vi "RTHeader.vi"(0 "Comment":string, 1 "Digitizer Settings":T10={"Digitizer delay (us) "=0.0, "rf points per line"=2048, "lines per plane"=128, "Samp Rate (Hz)"=100000000.0, "Additional dig delay (us)"=0.0, "Voltage Scale"=0.4, "Pre-Looks"=0, "Offset delay (us)"=0.0, "bits A/D"=8, "Avg Num"=1, "DigTimeOut"=5.0, "Rel Dig Delay"=0.0, "Dig Ch"=0, "LeCroyCluster"={"LeCroy Channels"=[TRUE, FALSE, FALSE, FALSE], "LC read pt offset"=0.0, "Sweep Avg"=FALSE}, "Main Digitizer"=enum."NI Digitizer", "Dig Config"=enum."Single channel", "Digitizer ID Cluster"={"Acqiris/Alazar/SP ID"=[], "NI Instr Handles"=[], "LeCroy VISA"="", "GaGe Handle"={"Handle"=0, "Sample size"=0, "Resolution"=0, "Offset"=0, "Channels"=0, "Boards"=0}, "ATS Ref"="ATS9350", "Acqiris Address"=["PCI::INSTR0"], "ADQRef"=refnum, "adq_cu_ptr"=refnum}, "Trigger Settings"={"Trig Source"=1, "Trig Coupling"=0, "Trig Slope"=0, "Level (mV)"=1500.0}, "Bulk Acq"=FALSE, "Bulk Start Indexes"=[], "Data Ref RF"=refnum, "NI ID/Channel"=[], "Total Dig CH"=1, "Xtra Ann Trig delay (us)"=10.0, "Fix Z Delay?"=FALSE, "One Way Transmission?"=FALSE, "Data Ref Log"=refnum} {"Trigger Settings"."Trig Slope" items=["Positive", "Negative"]; "Trigger Settings"."Level (mV)" format="%.2f"; "Trigger Settings"."Trig Coupling" items=["DC 1 MOhm", "AC 1 MOhm", "DC 50 Ohm", "AC 50 Ohm"]; "Trigger Settings"."Trig Source" items=["Chan 1", "External"]; "Rel Dig Delay" format="%.2f"; "DigTimeOut" format="%.2f"; "Avg Num" min=1; "Offset delay (us)" format="%.2f"; "Additional dig delay (us)" format="%.2f"; "Digitizer delay (us)" format="%.2f"}, 3 "Dig Word Size":u16=8, 5 "File Name In":string, 7 "Patient Info":T1={"Eye Selector"=enum."Right", "Plane"=1, "First Name"="", "Last Name"="", "Notes"="", "Patient ID"="", "Scan Location"=enum."Radio Selection 1"} {"Plane" min=1 max=12 step=1 scale=0.0..12.0}, 9 "Ann Array Params":T2={"Synth Foc?"=FALSE, "Focal Zones"=41, "Switch T/R"=0, "Trans Geometry (mm)"={"Transducer"=0, "Geo Focus"=12.0, "a (radius)"=3.0, "# of rings"=5, "kerf space "=0.1, "Center Freq"=12.0}, "Sub Ap Excite?"=FALSE, "Full Array Scan?"=FALSE, "Xmt/Rcv"={"XMIT"=[TRUE, TRUE, TRUE, TRUE, TRUE], "RCV"=[TRUE, TRUE, TRUE, TRUE, TRUE]}, "PulseSpacing (us)"=0.0, "Xmit Ring"=0, "XMIT CHS"=0, "RCV CHS"=0, "GPU?"=FALSE, "Save TIFF?"=FALSE, "downfactor"=1, "RCV 1CH"=0} {"RCV 1CH" items=["All", "1", "2", "3", "4", "5"]; "Trans Geometry (mm)"."Transducer" items=["6D 12R 40 MHz"=0, "10D 31R 20 MHz"=1, "10D 23R 20 MHz"=2, "6D 23R 40 MHz"=3, "4.5D 10.7R 40 MHz"=4, "9D 23.5R 20 MHz"=5, "9D 25.8R 20MHz"=6, "Enter"=99]; "Switch T/R" min=1 max=5 step=1}, 11 "Votage scaling":T15, 12 "Pulser Channel":i32, 14 "Scan Info":T5, 15 "Motion Settings":T6={"No Motion?"=FALSE, "Motion System"=enum."NI 735x", "Motion Bd ID"=1, "Motion Profile"="SMAC1", "# Axis"=1, "Reverse Z axis?"=TRUE, "SMAC Axis"=0, "scan pair"=enum."y-(x) scan", "RT fps"=6.0, "Steps per mm"=[1000, 1000, 1000, 1000], "Motor Parameters"={"velocity ct/s"=[10000.0, 10000.0, 10000.0, 50000.0], "accel ct/s^2"=[50000.0, 50000.0, 50000.0, 200000.0]}, "One Way Scan"=FALSE, "Reverse One Way Scan"=FALSE, "Global Position (mm)"=[], "Plane"=0, "Distance between\nscan lines (um)"=0.0, "Distance between\nscan planes (um)"=0.0, "number of scan planes"=1, "Total steps in line"=0, "Xtra plane\ndistance  (um)"=100, "Xtra planes "=1, "Add Axis"=FALSE, "overshoot cts"=200, "BKPT Shift"=0, "Scan Start Time (ms)"=0, "ESP VISA"="GPIB::1::INSTR", "3rd Axis"=1, "GL Ref Out"=refnum, "Galil Address"=""} {"3rd Axis" items=["x", "y", "z", "w"]; "Xtra planes" min=1; "Xtra plane\ndistance  (um)" min=0; "Distance between\nscan planes (um)" format="%.2f"; "Distance between\nscan lines (um)" format="%.2f"; "SMAC Axis" items=["None"=0, "Axis 1"=1, "Axis 2"=2, "Axis 3"=3, "Axis 4"=4, "Axis 5"=5, "Axis 6"=6, "Axis 7"=7, "Axis 8"=8, "Vector Space 1"=17, "Vector Space 2"=18, "Vector Space 3"=19, "Vector Space 4"=20]; "Motion Bd ID" min=1 max=32 step=1}) -> (4 "Header String Out":string, 10 "Header Out":T14={"header info"={"Header"="", "Head length"=0}, "A/D info"={"# rf points per line"=0, "# lines per scan"=0, "sample rate MHz"=0, "# A/D bits"=0, "# bytes per A/D"=0, "TGC Flag"=0, "A/D Type"=""}, "Tranducer Info"={"bandwidth"=0.0, "center freq"=0.0, "start freq"=0.0, "ID"=0}, "Scan Info"={"delay"=0.0, "pivot distance"=0.0, "sector scan angle"=0.0, "operator"="", "Scan Mode"="", "location"=""}, "Time/Date Info"={"date"="", "time"=""}, "RF Info"={"RF file name"="", "RF file att"="", "RF cal file name"="", "RF cal file att"=""}, "Patient Info"={"ID"="", "extended ID"="", "age"=0, "sex"="", "previously\nscanned"="", "PSA"=0.0, "LOS"=1, "Ethnicty 2"=3, "Race"=3}, "Tissue Type"={"organ"=0, "disease type"=0, "disease location"=0, "IQ_pts"=0, "RcvBuffer"=0, "RcvFrame"=0, "IQBuff"=0, "IQFrame"=0, "IQPage"=0}, "Votage scaling"={"Digitizer (dB)"=0.0, "Gain (dB)"=0.0, "Atten (dB)"=0.0}, "Comment"="", "Misc Info"={"avg num"=0, "c speed"=0, "Div By or SF zones"=0, "XMIT CHS"=0, "RCV CHS"=0, "Xmit angle"=0.0}, "Therapy Parameters"={"Theraputic Freq (MHz)"=0.1, "Time on (s)"=1.0, "Therapy amplitude (mV)"=50.0, "Lines Before"=20, "Lines After"=80}, "Scan Settings"={"Energy (uJ or V)"=0, "Damp (Ohm) or Fc"=0, "HP Filt (KHz)"=0, "LP Filt (MHz)"=0, "Gain (db)"=0, "prf (kHz)"=0.0, "Distance between\nscan lines (um)"=0, "Distance between\nscan planes (um)"=0, "Scan line gap (um)"=0.0, "Scan plane gap (um)"=0.0}, "Compression Parameters"={"F1 (MHz)"=0.0, "F2 (MHz)"=0.0, "% taper"=0.0, "duration"=0.0}, "Patient Info Xtra"={"First Name"="", "Last Name"="", "Notes"=""}, "ROI Box"=[]} {"Compression Parameters"."% taper" min=50 max=1000 format="%.2f"; "Compression Parameters"."F2 (MHz)" format="%.3f"; "Compression Parameters"."F1 (MHz)" format="%.3f"; "Scan Settings"."prf (kHz)" format="%.2f"; "Therapy Parameters"."Therapy amplitude (mV)" min=50 max=1000 format="%.2f"; "Therapy Parameters"."Time on (s)" format="%.3f"; "Therapy Parameters"."Theraputic Freq (MHz)" format="%.3f"; "Patient Info"."Race" items=["Am Ind or Alaska", "Asian", "Hawaiian, Pac Isl", "Black or Afr Amer", "White", "more than one race", "unknown"]; "Patient Info"."Ethnicty 2" items=["Hispanic", "Non-Hispanic", "unknown"]; "Patient Info"."LOS" items=["1", "2", "3", "4", "5"]; "Patient Info"."PSA" format="%.1f"; "Scan Info"."delay" format="%.2f"; "Scan Info"."pivot distance" format="%.2f"; "Scan Info"."sector scan angle" format="%.2f"; "Tranducer Info"."bandwidth" format="%.2f"; "Tranducer Info"."center freq" format="%.2f"; "Tranducer Info"."start freq" format="%.2f"})   [LabVIEW 2022 SP3]
uses:
  ViewData/-ReadEye/Header.ctl
  ScanningControl/Digitizers/-DigitizerRoutines/DigitizerSettings.ctl
  ScanningControl/Digitizers/-DigitizerRoutines/Digitizer.ctl
  ScanningControl/Digitizers/-DigitizerRoutines/DigConfig.ctl
  ScanningControl/Digitizers/-DigitizerRoutines/DigitizerID.ctl
  C:/Windows/System32/ADQAPI_dotNet_helper.dll
  ScanningControl/Motion Controllers/NI_controller/-NI_MotionRoutines/MotionParameters.ctl
  ScanningControl/Motion Controllers/NI_controller/-NI_MotionRoutines/MotionSys.ctl
  ScanningControl/Motion Controllers/-MotionRoutines/ScanAxis.ctl
  ScanningControl/Motion Controllers/-MotionRoutines/3rdAxis.ctl
  Annular Array/-AnnularRoutines/AnnularArray.ctl
  Annular Array/-AnnularRoutines/TransGeometry.ctl
  Annular Array/-AnnularRoutines/ArrayGeometry.ctl
  PatientInfoDef.ctl
  ScanningControl/Motion Controllers/-MotionRoutines/MotionGlobals.vi
  ScanningControl/Pulsers/PulserGlobals.vi
  Patient Routines/PatientGlobals.vi
  ScanningControl/Switch Modules/SwitchGlobals.vi
panel:
  # "1-D and 2-D B scan settings"
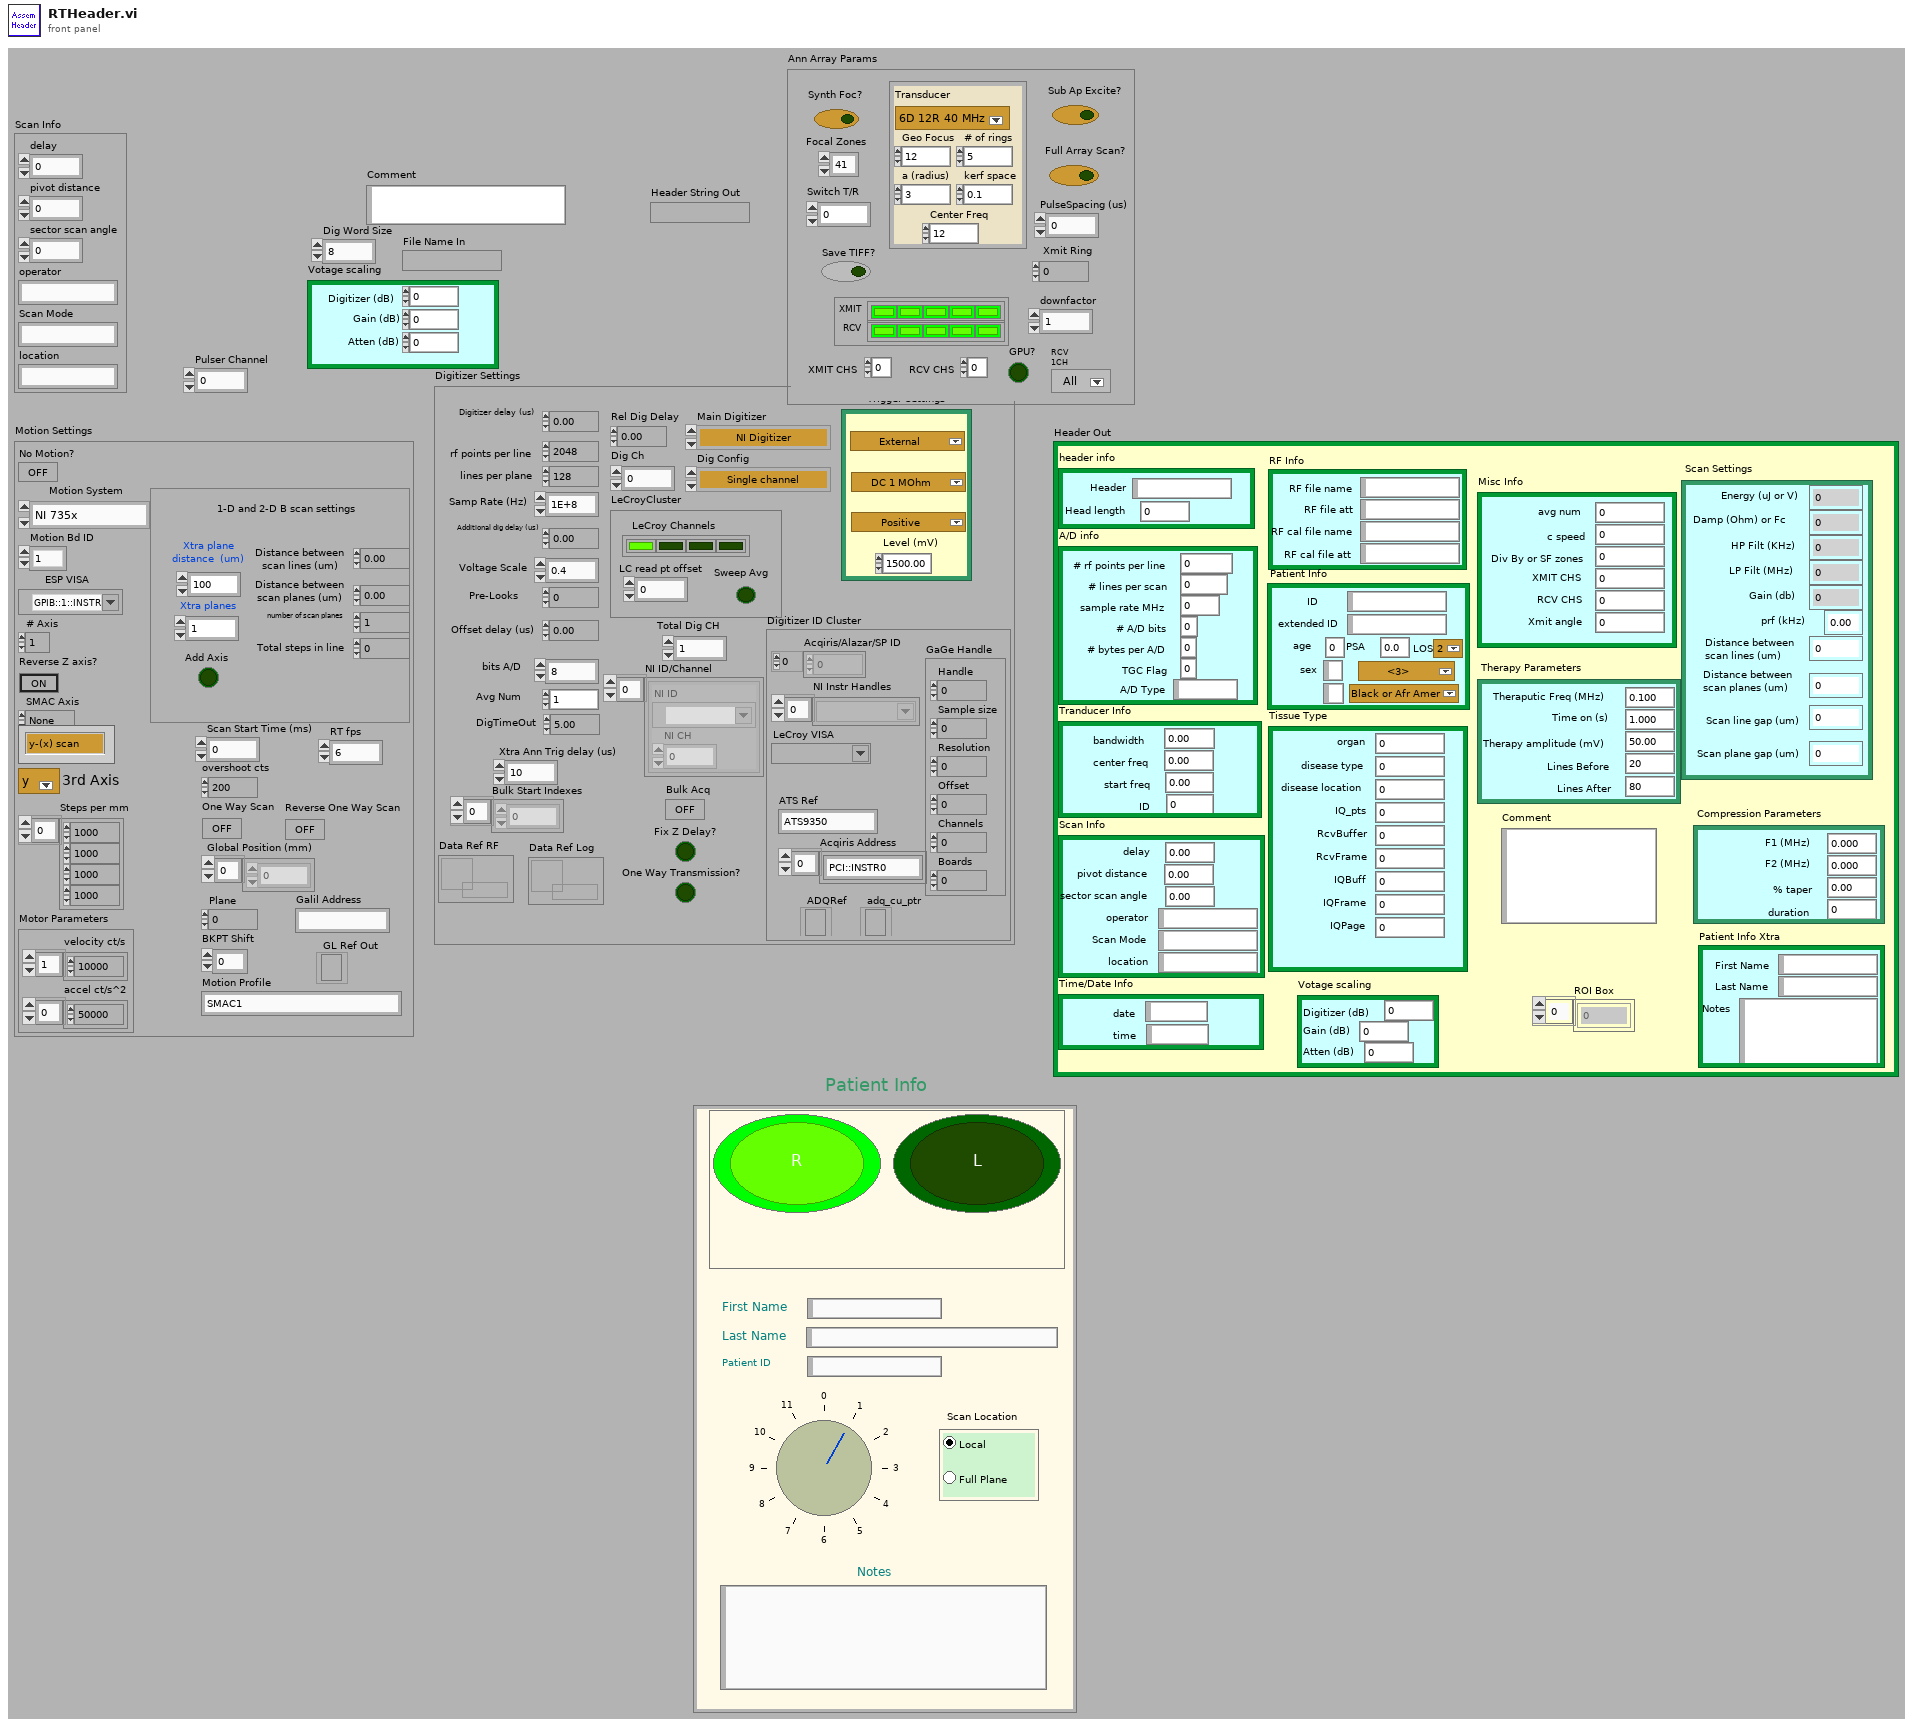
[diagram p1: front panel]
types:
  T1 = typedef "PatientInfoDef.ctl" = cluster{"Eye Selector":enum32{"Left", "Right"}, "Plane":i8, "First Name":string, "Last Name":string, "Notes":string, "Patient ID":string, "Scan Location":enum32{"Radio Selection 1", "Radio Selection 2"}}
  T2 = typedef "AnnularArray.ctl" = cluster{"Synth Foc?":bool, "Focal Zones":i16, "Switch T/R":i16, "Trans Geometry (mm)":T3, "Sub Ap Excite?":bool, "Full Array Scan?":bool, "Xmt/Rcv":cluster{"XMIT":bool[], "RCV":bool[]}, "PulseSpacing (us)":sgl, "Xmit Ring":i32, "XMIT CHS":u8, "RCV CHS":u8, "GPU?":bool, "Save TIFF?":bool, "downfactor":i32, "RCV 1CH":u16}
  T3 = typedef "TransGeometry.ctl" = cluster{"Transducer":T4, "Geo Focus":dbl, "a (radius)":dbl, "# of rings":i32, "kerf space ":dbl, "Center Freq":dbl}
  T4 = typedef "ArrayGeometry.ctl" = u16
  T5 = cluster{"delay":sgl, "pivot distance":sgl, "sector scan angle":sgl, "operator":string, "Scan Mode":string, "location":string}
  T6 = typedef "MotionParameters.ctl" = cluster{"No Motion?":bool, "Motion System":T7, "Motion Bd ID":u8, "Motion Profile":string, "# Axis":i8, "Reverse Z axis?":bool, "SMAC Axis":u16, "scan pair":T8, "RT fps":sgl, "Steps per mm":i32[], "Motor Parameters":cluster{"velocity ct/s":dbl[], "accel ct/s^2":dbl[]}, "One Way Scan":bool, "Reverse One Way Scan":bool, "Global Position (mm)":dbl[], "Plane":i32, "Distance between\nscan lines (um)":sgl, "Distance between\nscan planes (um)":sgl, "number of scan planes":i32, "Total steps in line":i32, "Xtra plane\ndistance  (um)":i32, "Xtra planes ":i32, "Add Axis":bool, "overshoot cts":i32, "BKPT Shift":i32, "Scan Start Time (ms)":u32, "ESP VISA":refnum<visa-resource-name>, "3rd Axis":T9, "GL Ref Out":refnum<k7>, "Galil Address":string}
  T7 = typedef "MotionSys.ctl" = enum16{"MM3000", "NI 735x", "Newport ESP", "No Motion Card", "Galil"}
  T8 = typedef "ScanAxis.ctl" = enum16{"y-(x) scan", "x-(y) scan", "z-(x) scan", "z-(y) scan", "y-(z) scan", "x-(z) scan", "w-(x) scan", "w-(y) scan", "w-(z) scan", "x-(w) scan", "y-(w) scan", "z-(w) scan"}
  T9 = typedef "3rdAxis.ctl" = u16
  T10 = typedef "DigitizerSettings.ctl" = cluster{"Digitizer delay (us) ":dbl, "rf points per line":i32, "lines per plane":i32, "Samp Rate (Hz)":dbl, "Additional dig delay (us)":dbl, "Voltage Scale":dbl, "Pre-Looks":i32, "Offset delay (us)":dbl, "bits A/D":i8, "Avg Num":i32, "DigTimeOut":sgl, "Rel Dig Delay":sgl, "Dig Ch":i32, "LeCroyCluster":cluster{"LeCroy Channels":bool[], "LC read pt offset":dbl, "Sweep Avg":bool}, "Main Digitizer":T11, "Dig Config":T12, "Digitizer ID Cluster":T13, "Trigger Settings":cluster{"Trig Source":u16, "Trig Coupling":u16, "Trig Slope":u16, "Level (mV)":dbl}, "Bulk Acq":bool, "Bulk Start Indexes":i32[], "Data Ref RF":refnum<data-value>, "NI ID/Channel":cluster{"NI ID":refnum<k15>, "NI CH":i32}[], "Total Dig CH":i32, "Xtra Ann Trig delay (us)":dbl, "Fix Z Delay?":bool, "One Way Transmission?":bool, "Data Ref Log":refnum<data-value>}
  T11 = typedef "Digitizer.ctl" = enum16{"Acqiris Digitizer", "NI Digitizer", "LeCroy", "GaGe", "AlazarTech", "No Digitizer", "Teledyne"}
  T12 = typedef "DigConfig.ctl" = enum16{"Single channel", "2 Chans w/ 2 Acqiris", "2 Chans w/ 1 Acqiris", "5-CH Pulser New", "5-CH pulser w/ ann array", "5-pass style ann array", "Empty"}
  T13 = typedef "DigitizerID.ctl" = cluster{"Acqiris/Alazar/SP ID":u32[], "NI Instr Handles":refnum<k15>[], "LeCroy VISA":refnum<visa-resource-name>, "GaGe Handle":cluster{"Handle":u32, "Sample size":u32, "Resolution":i32, "Offset":i32, "Channels":u32, "Boards":u32}, "ATS Ref":string, "Acqiris Address":string[], "ADQRef":refnum<k24>, "adq_cu_ptr":refnum<k24>}
  T14 = typedef "Header.ctl" = cluster{"header info":cluster{"Header":string, "Head length":i16}, "A/D info":cluster{"# rf points per line":u16, "# lines per scan":u16, "sample rate MHz":u16, "# A/D bits":i16, "# bytes per A/D":u16, "TGC Flag":u16, "A/D Type":string}, "Tranducer Info":cluster{"bandwidth":sgl, "center freq":sgl, "start freq":sgl, "ID":i32}, "Scan Info":cluster{"delay":sgl, "pivot distance":sgl, "sector scan angle":sgl, "operator":string, "Scan Mode":string, "location":string}, "Time/Date Info":cluster{"date":string, "time":string}, "RF Info":cluster{"RF file name":string, "RF file att":string, "RF cal file name":string, "RF cal file att":string}, "Patient Info":cluster{"ID":string, "extended ID":string, "age":u16, "sex":string, "previously\nscanned":string, "PSA":sgl, "LOS":u8, "Ethnicty 2":u8, "Race":u8}, "Tissue Type":cluster{"organ":i16, "disease type":i16, "disease location":i16, "IQ_pts":u16, "RcvBuffer":u8, "RcvFrame":u16, "IQBuff":u8, "IQFrame":u16, "IQPage":u8}, "Votage scaling":cluster{"Digitizer (dB)":sgl, "Gain (dB)":sgl, "Atten (dB)":sgl}, "Comment":string, "Misc Info":cluster{"avg num":u16, "c speed":i16, "Div By or SF zones":i16, "XMIT CHS":u8, "RCV CHS":u8, "Xmit angle":sgl}, "Therapy Parameters":cluster{"Theraputic Freq (MHz)":sgl, "Time on (s)":sgl, "Therapy amplitude (mV)":sgl, "Lines Before":u16, "Lines After":u16}, "Scan Settings":cluster{"Energy (uJ or V)":u8, "Damp (Ohm) or Fc":u8, "HP Filt (KHz)":u8, "LP Filt (MHz)":u8, "Gain (db)":u8, "prf (kHz)":sgl, "Distance between\nscan lines (um)":u16, "Distance between\nscan planes (um)":u16, "Scan line gap (um)":sgl, "Scan plane gap (um)":sgl}, "Compression Parameters":cluster{"F1 (MHz)":sgl, "F2 (MHz)":sgl, "% taper":sgl, "duration":sgl}, "Patient Info Xtra":cluster{"First Name":string, "Last Name":string, "Notes":string}, "ROI Box":u16[]}
  T15 = cluster{"Digitizer (dB)":sgl, "Gain (dB)":sgl, "Atten (dB)":sgl}
  T16 = typedef "location.ctl" = enum16{"Automatic", "WCM Main", "Hawaii", "Columbia MM3000", "Columbia  NI System", "NYU", "RRI 2", "UHI Allen", "CUMC RT", "Chiba", "Stony Brook", "WCM Microscopy", "WCM Aeoretch", "WCM Optics Lab", "WCM Main 2Axis", "WCM Rotation", "WCM SAM SMAC", "SERI GP"}
  T17 = typedef "ScanType2.ctl" = enum16{"Therapy With Scan", "M scan", "M Scan With Therapy Burst", "1-D B Scan", "1-D B Scan With Therapy Burst", "2-D B Scan", "2-D B Scan With Therapy Burst", "Rotational Scan", "1-D B-Scan PRF", "2-D B-Scan PRF", "Real-Time Scan", "Contrast Agents", "1-D w/ Real-Time Set Up", "Dual Transducer", "Acoustic Microscopy", "Hydrophone Scanning"}
  T18 = cluster{"# rf points per line":u16, "# lines per scan":u16, "sample rate MHz":u16, "# A/D bits":i16, "# bytes per A/D":u16, "TGC Flag":u16, "A/D Type":string}
  T19 = cluster{"bandwidth":sgl, "center freq":sgl, "start freq":sgl, "ID":i32}
  T20 = cluster{"Energy (uJ or V)":u8, "Damp (Ohm) or Fc":u8, "HP Filt (KHz)":u8, "LP Filt (MHz)":u8, "Gain (db)":u8, "prf (kHz)":sgl, "Distance between\nscan lines (um)":u16, "Distance between\nscan planes (um)":u16, "Scan line gap (um)":sgl, "Scan plane gap (um)":sgl}
  T21 = typedef "pulser.ctl" = enum16{"Pan 5900", "Daxsonics", "Agilent 33xxx", "UTEX", "JSR", "WMC Mono-Cycle", "No Pulser", "NYU AVTECH", "Tabor W1281A", "Pan 5800", "Unlisted", "Tabor WX2182B"}
  T22 = cluster{"Energy (microJ)":u8, "Damping (In Ohm)":u8, "HP Filt(KHz) ":u16, "LP Filt (MHz)":u8, "Gain (db)":u8, "Atten (dB)":sgl}
  T23 = typedef "UTEX Controls.ctl" = cluster{"High Pass On":bool, "High Pass Filter (MHz)":i16, "Low Pass On":bool, "Low Pass Filter (MHz)":i16, "PE Gain (dB)":i16, "Voltage":i16, "Pulse Width (ns)":dbl, "Mode":bool, "PC Gain (dB)":i16, "Trig Source":bool, "Rep Rate (Hz)":i16, "PULSE":bool}
  T24 = cluster{"F1 (MHz)":sgl, "F2 (MHz)":sgl, "Tukey taper":sgl, "duration":sgl}
  T25 = cluster{"RF file name":string, "RF file att":string, "RF cal file name":string, "RF cal file att":string}
  T26 = cluster{"ID":string, "extended ID":string, "age":u16, "sex":string, "previously\nscanned":string, "PSA":sgl, "LOS":u8, "Ethnicty 2":u8, "Race":u8}
  T27 = cluster{"organ":i16, "disease type":i16, "disease location":i16, "IQ_pts":u16, "RcvBuffer":u8, "RcvFrame":u16, "IQBuff":u8, "IQFrame":u16, "IQPage":u8}
  T28 = cluster{"avg num":u16, "c speed":i16, "Div By or SF zones":i16, "XMIT CHS":u8, "RCV CHS":u8, "Xmit angle":sgl}
  T29 = cluster{"Therapy frequency (MHz)":dbl, "Therapy amplitude (mV)":dbl, "time therapy on (s)":dbl, "Therapy Delay (ms) ":dbl, "Time (s)":dbl}
  T30 = cluster{"Theraputic Freq (MHz)":sgl, "Time on (s)":sgl, "Therapy amplitude (mV)":sgl, "Lines Before":u16, "Lines After":u16}
  T31 = typedef "LymphNodeInfo.ctl" = cluster{"Patient Number":u32, "Node Set":string, "Node Number":u32, "Tissue Type":T32, "Tissue Location (Other)":string, "Node Classification":enum16{"Whole Node", "Piece A", "Piece B", "Piece C"}, "Fresh?":enum32{"Fresh?", "Fixed?", "Refrigerated?"}, "Year":u32}
  T32 = typedef "TissueTypeScan.ctl" = enum16{"Breast", "Gastric", "Stomach", "Rectal", "Colon", "Head & Neck", "Other"}
  T33 = cluster{"First Name":string, "Last Name":string, "Notes":string}
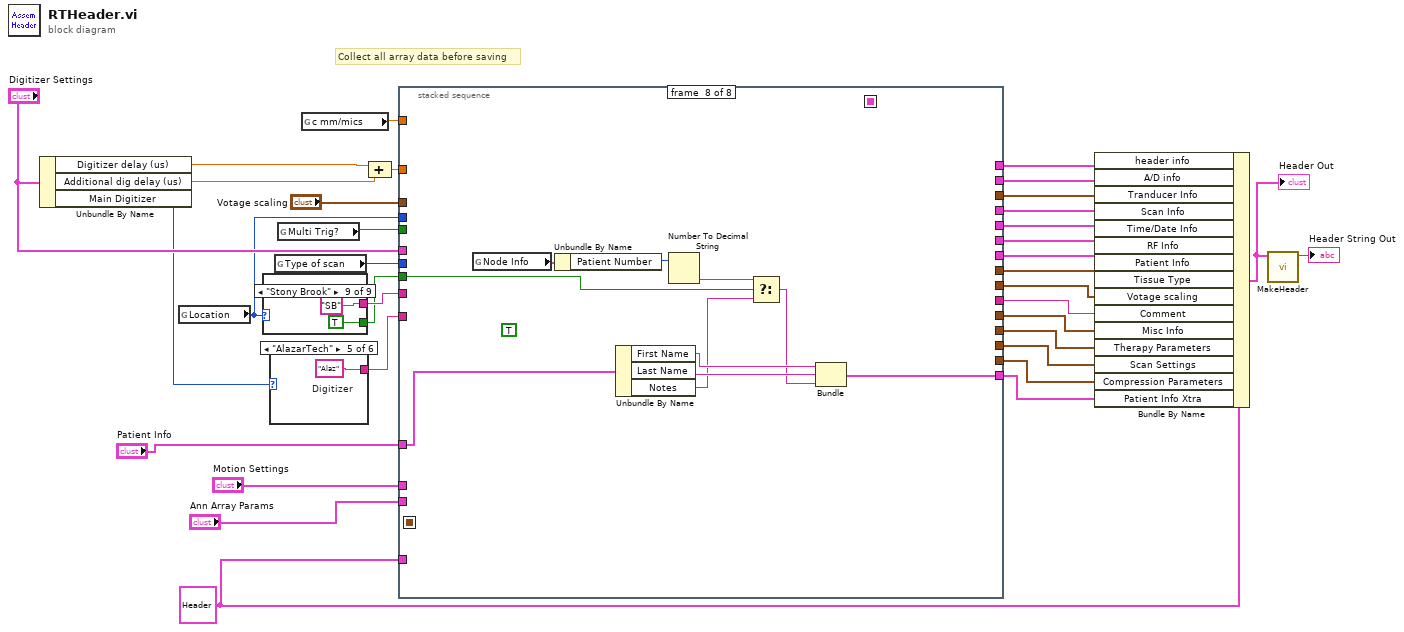
[diagram p0: block diagram]
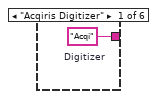
[diagram p2: hidden frame]
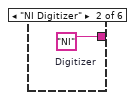
[diagram p3: hidden frame]
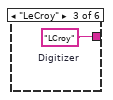
[diagram p4: hidden frame]
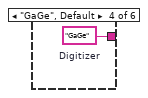
[diagram p5: hidden frame]
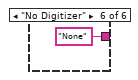
[diagram p6: hidden frame]
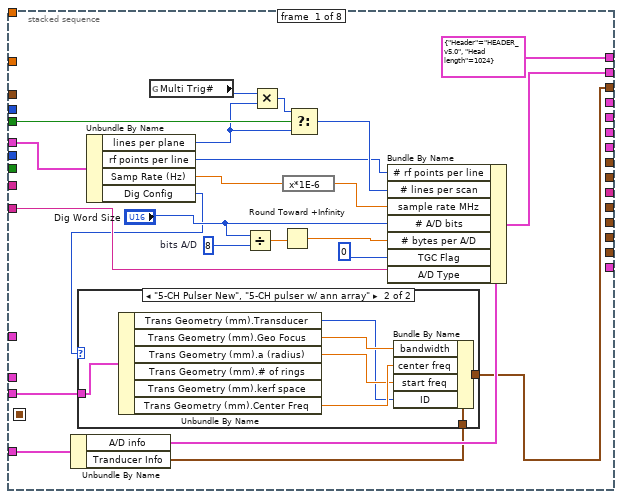
[diagram p7: hidden frame]
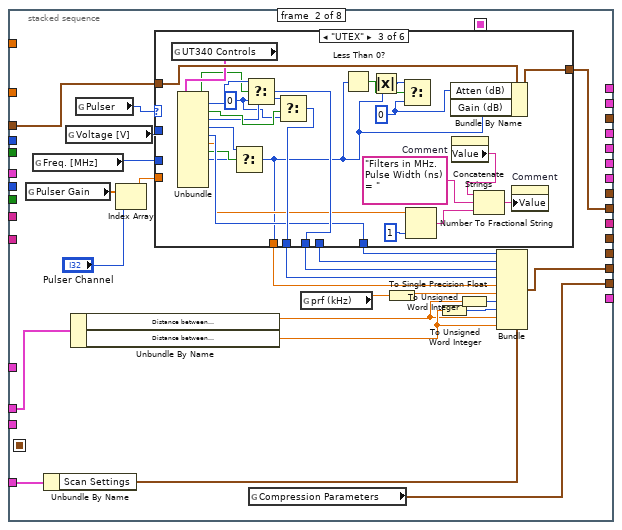
[diagram p9: hidden frame]
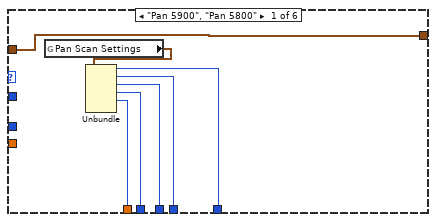
[diagram p10: hidden frame]
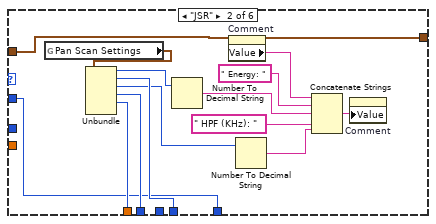
[diagram p11: hidden frame]
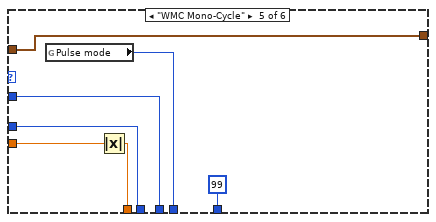
[diagram p13: hidden frame]
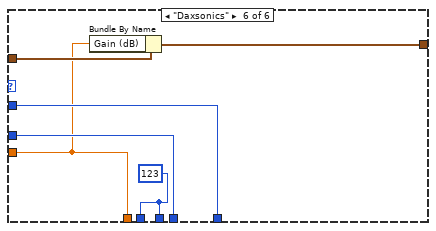
[diagram p14: hidden frame]
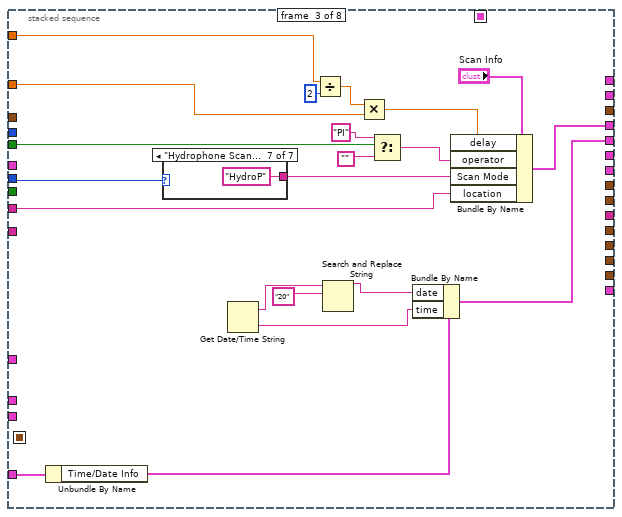
[diagram p15: hidden frame]
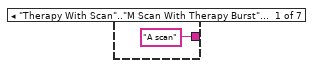
[diagram p16: hidden frame]
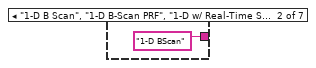
[diagram p17: hidden frame]
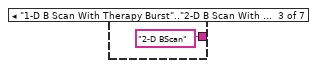
[diagram p18: hidden frame]
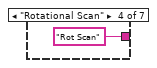
[diagram p19: hidden frame]
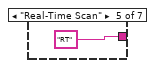
[diagram p20: hidden frame]
diagram:
  w12 = T14 {"header info"={"Header"="", "Head length"=0}, "A/D info"={"# rf points per line"=0, "# lines per scan"=0, "sample rate MHz"=0, "# A/D bits"=0, "# bytes per A/D"=0, "TGC Flag"=0, "A/D Type"=""}, "Tranducer Info"={"bandwidth"=0.0, "center freq"=0.0, "start freq"=0.0, "ID"=0}, "Scan Info"={"delay"=0.0, "pivot distance"=0.0, "sector scan angle"=0.0, "operator"="", "Scan Mode"="", "location"=""}, "Time/Date Info"={"date"="", "time"=""}, "RF Info"={"RF file name"="", "RF file att"="", "RF cal file name"="", "RF cal file att"=""}, "Patient Info"={"ID"="", "extended ID"="", "age"=0, "sex"="", "previously\nscanned"="", "PSA"=0.0, "LOS"=1, "Ethnicty 2"=3, "Race"=3}, "Tissue Type"={"organ"=0, "disease type"=0, "disease location"=0, "IQ_pts"=0, "RcvBuffer"=0, "RcvFrame"=0, "IQBuff"=0, "IQFrame"=0, "IQPage"=0}, "Votage scaling"={"Digitizer (dB)"=0.0, "Gain (dB)"=0.0, "Atten (dB)"=0.0}, "Comment"="", "Misc Info"={"avg num"=0, "c speed"=0, "Div By or SF zones"=0, "XMIT CHS"=0, "RCV CHS"=0, "Xmit angle"=0.0}, "Therapy Parameters"={"Theraputic Freq (MHz)"=0.0, "Time on (s)"=0.0, "Therapy amplitude (mV)"=0.0, "Lines Before"=0, "Lines After"=0}, "Scan Settings"={"Energy (uJ or V)"=0, "Damp (Ohm) or Fc"=0, "HP Filt (KHz)"=0, "LP Filt (MHz)"=0, "Gain (db)"=0, "prf (kHz)"=0.0, "Distance between\nscan lines (um)"=0, "Distance between\nscan planes (um)"=0, "Scan line gap (um)"=0.0, "Scan plane gap (um)"=0.0}, "Compression Parameters"={"F1 (MHz)"=0.0, "F2 (MHz)"=0.0, "% taper"=0.0, "duration"=0.0}, "Patient Info Xtra"={"First Name"="", "Last Name"="", "Notes"=""}, "ROI Box"=[0, 0, 0, 0]} ("Header In")
  # "Collect all array data before saving"
  n1 = Unbundle By Name("Digitizer Settings") -> ("Digitizer delay (us)"=w16:dbl, "Additional dig delay (us)"=w15:dbl, "Main Digitizer"=w13:T11)
  n2 = global read "MotionGlobals.vi" "Location"() -> (w4:T16)
  n3 = case shown="\"Stony Brook\"" w4 {
    tunnel: ["RRI" "HI" "WMC" "WMC" "NYU" "UHI" "CU" "JP" "SB"] -> w32
    tunnel: [FALSE TRUE FALSE FALSE FALSE FALSE FALSE FALSE TRUE] -> w3
    frame "WCM Main", Default {
    }
    frame "Hawaii" {
    }
    frame "Columbia MM3000" {
    }
    frame "Columbia  NI System" {
    }
    frame "NYU" {
    }
    frame "UHI Allen" {
    }
    frame "CUMC RT" {
    }
    frame "Chiba" {
    }
    frame "Stony Brook" {
    }
  }
  n4 = case shown="\"AlazarTech\"" w13 {
    tunnel: [w53 w54 w55 w56 w57 "None" ("Digitizer")] -> w17
    frame "Acqiris Digitizer" {
      w53 = "Acqi"  # Digitizer
    }
    frame "NI Digitizer" {
      w54 = "NI"  # Digitizer
    }
    frame "LeCroy" {
      w55 = "LCroy"  # Digitizer
    }
    frame "GaGe", Default {
      w56 = "GaGe"  # Digitizer
    }
    frame "AlazarTech" {
      w57 = "Alaz"  # Digitizer
    }
    frame "No Digitizer" {
    }
  }
  n5 = global read "MotionGlobals.vi" "Type of scan"() -> (w5:T17)
  n6 = global read "MotionGlobals.vi" "Multi Trig?"() -> (w21:bool)
  n7 = global read "MotionGlobals.vi" "c mm/mics"() -> (w29:sgl)
  n8 = Compound Arithmetic op=ADD(w16, w15) -> (w24:dbl)
  n9 = stacked-sequence {
    seq-local: [_ _ _ _ w226 _ _ _] -> [_ _ _ _ _ w261 _ _]
    seq-local: [_ _ _ w201 _ _ _ _] -> [_ _ _ _ _ w259 _ _]
    tunnel: [cluster{"Header":string, "Head length":i16} {"Header"="HEADER_v5.0", "Head length"=1024} ("header info") _ _ _ _ _ _ _] -> w34
    tunnel: [w77 _ _ _ _ _ _ _] -> w33
    tunnel: w32 -> [_ _ w188 _ _ _ _ _]
    tunnel: [_ _ w189 _ _ _ _ _] -> w31
    tunnel: w17 -> [w76 _ _ _ _ _ _ _]
    tunnel: [w61 _ _ _ _ _ _ _] -> w30
    tunnel: w29 -> [_ _ w187 _ w240 _ _ _]
    tunnel: [_ _ w182 _ _ _ _ _] -> w28
    tunnel: "Votage scaling" -> [_ w101 _ w207 _ _ _ _]
    tunnel: [_ _ _ w209 _ _ _ _] -> w25
    tunnel: w24 -> [_ _ w178 _ _ _ _ _]
    tunnel: [_ _ _ _ _ w258 _ _] -> w23
    tunnel: [_ w92 _ _ _ _ _ _] -> w7
    tunnel: [_ _ _ _ w225 _ _ _] -> w22
    tunnel: [_ _ _ _ "Comment" _ _ _] -> w8
    tunnel: w21 -> [w74 _ w177 _ _ _ _ _]
    tunnel: [_ _ _ _ _ w260 _ _] -> w9
    tunnel: [_ _ _ _ _ _ w302 _] -> w10
    tunnel: [_ w105 _ _ _ _ _ _] -> w11
    tunnel: [_ w104 _ _ _ _ _ _] -> w20
    tunnel: [_ _ _ _ _ _ _ w310] -> w18
    tunnel: "Patient Info" -> [_ _ _ _ w232 _ _ w309]
    tunnel: "Digitizer Settings" -> [w67 _ _ _ w231 _ w301 _]
    tunnel: w12 -> [w64 w95 w176 w204 w229 _ w295 _]
    tunnel: "Motion Settings" -> [_ w93 _ _ _ w267 _ _]
    tunnel: w5 -> [_ _ w173 _ _ w254 _ _]
    tunnel: w4 -> [_ _ _ _ _ _ _ _]
    tunnel: w3 -> [_ _ _ _ _ _ _ w304]
    tunnel: "Ann Array Params" -> [w59 _ _ _ w220 _ _ _]
    frame #0 {
      w79 = 8  # bits A/D
      n10 = Unbundle By Name(w64) -> ("A/D info"=w63:T18, "Tranducer Info"=w62:T19)
      n11 = Unbundle By Name(w67) -> ("lines per plane"=w65:i32, "rf points per line"=w66:i32, "Samp Rate (Hz)"=w68:dbl, "Dig Config"=w60:T12)
      n12 = case shown="\"5-CH Pulser New\", \"5-CH pulser w/ ann array\"" w60 {
        tunnel: w62 -> [w82 w89]
        tunnel: [w82 w88] -> w61
        tunnel: w59 -> [_ w83]
        frame "Single channel", Default {
        }
        frame "5-CH Pulser New", "5-CH pulser w/ ann array" {
          n13 = Unbundle By Name(w83) -> ("Trans Geometry (mm).Transducer"=w84:T4, "Trans Geometry (mm).Geo Focus"=w86:dbl, "Trans Geometry (mm).a (radius)"=w85:dbl, "Trans Geometry (mm).Center Freq"=w87:dbl)  [unwired: 2 out]
          n14 = Bundle By Name(cluster=w89, "bandwidth"=w86, "center freq"=w87, "start freq"=w85, "ID"=w84) -> (w88:T19)
        }
      }
      n15 = global read "MotionGlobals.vi" "Multi Trig#"() -> (w70:i32)
      n16 = Divide(x="Dig Word Size", y=w79) -> (x/y=w80:dbl)
      n17 = Multiply(x=w70, y=w65) -> (x*y=w69:i32)
      n18 = Round Toward +Infinity(x=w80) -> (ceil(x): smallest int >= x=w78:dbl)
      n19 = expression code="x*1E-6"(w68) -> (w73:dbl)
      n20 = Select(t=w69, s=w74, f=w65) -> (s? t:f=w71:i32)
      n21 = Bundle By Name(cluster=w63, "# rf points per line"=w66, "# lines per scan"=w71, "sample rate MHz"=w73, "# A/D bits"="Dig Word Size", "# bytes per A/D"=w78, "TGC Flag"=u16 0, "A/D Type"=w76) -> (w77:T18)
    }
    frame #1 {
      n22 = global read "PulserGlobals.vi" "Pulser Gain"() -> (w97:sgl[])
      n23 = global read "PulserGlobals.vi" "Freq. [MHz]"() -> (w98:i16)
      n24 = Unbundle By Name(w95) -> ("Scan Settings"=w94:T20)
      n25 = global read "PulserGlobals.vi" "Voltage [V]"() -> (w99:i16)
      n26 = Unbundle By Name(w93) -> ("Distance between\nscan lines (um)"=w90:sgl, "Distance between\nscan planes (um)"=w91:sgl)
      n27 = global read "PulserGlobals.vi" "Pulser"() -> (w100:T21)
      n28 = Index Array(array=w97, index="Pulser Channel") -> (element=w103:sgl)
      n29 = case shown="\"UTEX\"" w100 {
        tunnel: [w120 w129 w147 _ 99 w172] -> w110
        tunnel: [w119 w134 _ _ w160 w171] -> w109
        tunnel: [w118 _ w151 _ w164 w170] -> w108
        tunnel: [w117 w133 w148 _ w163 w170] -> w107
        tunnel: [w116 w132 w135 _ w165 w168] -> w106
        tunnel: w99 -> [_ w129 _ _ w164 w172]
        tunnel: w98 -> [_ _ _ _ w163 w171]
        tunnel: w103 -> [_ _ _ _ w162 w168]
        tunnel: w101 -> [w115 w131 w158 w159 w161 w169]
        tunnel: [w115 w131 w143 w159 w161 w167] -> w92
        frame "Pan 5900", "Pan 5800" {
          n30 = global read "PulserGlobals.vi" "Pan Scan Settings"() -> (w114:T22)
          n31 = Unbundle(w114) -> ("Energy (microJ)"=w120:u8, "Damping (In Ohm)"=w119:u8, "HP Filt(KHz)"=w118:u16, "LP Filt (MHz)"=w117:u8, "Gain (db)"=w116:u8)  [unwired: 1 out]
        }
        frame "JSR" {
          n32 = global read "PulserGlobals.vi" "Pan Scan Settings"() -> (w130:T22)
          n33 = Unbundle(w130) -> ("Energy (microJ)"=w121:u8, "Damping (In Ohm)"=w134:u8, "HP Filt(KHz)"=w122:u16, "LP Filt (MHz)"=w133:u8, "Gain (db)"=w132:u8)  [unwired: 1 out]
          n34 = Number To Decimal String(number=w121) -> (decimal integer string=w125:string)  [unwired: 1 in]
          n35 = property on="Comment" class="Str"() -> ("Value"=w127:string)  [unwired: 2 in, 2 out]
          n36 = Number To Decimal String(number=w122) -> (decimal integer string=w123:string)  [unwired: 1 in]
          n37 = Concatenate Strings(w127, " Energy: " ("string"), w125, " HPF (KHz): " ("string"), w123) -> (w128:string)
          n38 = property on="Comment" class="Str"("Value"=w128) -> ()  [unwired: 2 in, 2 out]
        }
        frame "UTEX" {
          w136 = i16 0 ("f")
          w138 = i16 0 ("f")
          n39 = global read "PulserGlobals.vi" "UT340 Controls"() -> (w155:T23)
          n40 = Unbundle(w155) -> ("High Pass On"=w152:bool, "High Pass Filter (MHz)"=w153:i16, "Low Pass On"=w150:bool, "Low Pass Filter (MHz)"=w149:i16, "PE Gain (dB)"=w144:i16, "Voltage"=w147:i16, "Pulse Width (ns)"=w140:dbl, "Mode"=w146:bool, "PC Gain (dB)"=w145:i16)  [unwired: 3 out]
          n41 = Select(t=w144, s=w146, f=w145) -> (s? t:f=w135:i16)
          n42 = Select(t=w153, s=w152, f=w138) -> (s? t:f=w151:i16)
          n43 = Select(t=w149, s=w150, f=w138) -> (s? t:f=w148:i16)
          n44 = Less Than 0?(x=w135) -> (x < 0?=w142:bool)
          n45 = Absolute Value(x=w135) -> (abs(x)=w141:i16)
          n46 = Select(t=w141, s=w142, f=w136) -> ()  [unwired: 1 out]
          n47 = Number To Fractional String(number=w140, precision (6)=i16 1 ("width (-)")) -> (F-format string=w139:string)  [unwired: 2 in]
          n48 = Bundle By Name(cluster=w158, "Atten (dB)"=w136, "Gain (dB)"=w135) -> (w143:T15)
          n49 = property on="Comment" class="Str"() -> ("Value"=w156:string)  [unwired: 2 in, 2 out]
          n50 = Concatenate Strings(w156, "Filters in MHz. Pulse Width (ns) = " ("string"), w139) -> (w157:string)
          n51 = property on="Comment" class="Str"("Value"=w157) -> ()  [unwired: 2 in, 2 out]
        }
        frame "Agilent 33xxx", Default {
        }
        frame "WMC Mono-Cycle" {
          n52 = global read "PulserGlobals.vi" "Pulse mode"() -> (w160:u16)
          n53 = Absolute Value(x=w162) -> (abs(x)=w165:sgl)
        }
        frame "Daxsonics" {
          w170 = 123
          n54 = Bundle By Name(cluster=w169, "Gain (dB)"=w168) -> (w167:T15)
        }
      }
      n55 = global read "MotionGlobals.vi" "Compression Parameters"() -> (w104:T24)
      n56 = global read "PulserGlobals.vi" "prf (kHz)"() -> (w96:dbl)
      n57 = To Single Precision Float(number=w96) -> (single precision float=w111:sgl)
      n58 = To Unsigned Word Integer(number=w91) -> (unsigned 16bit integer=w113:u16)
      n59 = To Unsigned Word Integer(number=w90) -> (unsigned 16bit integer=w112:u16)
      n60 = Bundle(cluster=w94, "Energy (uJ or V)"=w110, "Damp (Ohm) or Fc"=w109, "HP Filt (KHz)"=w108, "LP Filt (MHz)"=w107, "Gain (db)"=w106, "prf (kHz)"=w111, "Distance between\nscan lines (um)"=w112, "Distance between\nscan planes (um)"=w113, "Scan line gap (um)"=w90, "Scan plane gap (um)"=w91) -> (w105:T20)
    }
    frame #2 {
      n61 = Unbundle By Name(w176) -> ("Time/Date Info"=w175:cluster{"date":string, "time":string})
      n62 = case shown="\"Hydrophone Scanning\"" w173 {
        tunnel: ["A scan" "1-D BScan" "2-D BScan" "Rot Scan" "RT" "CA" "HydroP"] -> w183
        frame "Therapy With Scan".."M Scan With Therapy Burst", Default {
        }
        frame "1-D B Scan", "1-D B-Scan PRF", "1-D w/ Real-Time Set Up" {
        }
        frame "1-D B Scan With Therapy Burst".."2-D B Scan With Therapy Burst", "2-D B-Scan PRF" {
        }
        frame "Rotational Scan" {
        }
        frame "Real-Time Scan" {
        }
        frame "Contrast Agents" {
        }
        frame "Hydrophone Scanning" {
        }
      }
      n63 = Get Date/Time String() -> (date string=w192:string, time string=w191:string)  [unwired: 3 out]
      n64 = Divide(x=w187, y=2) -> (x/y=w186:sgl)
      n65 = Search and Replace String(input string=w192, search string="20") -> (result string=w190:string)  [unwired: 2 in, 7 out]
      n66 = Multiply(x=w186, y=w178) -> (x*y=w185:dbl)
      n67 = Select(t="PI", s=w177, f="") -> (s? t:f=w179:string)
      n68 = Bundle By Name(cluster=w175, "date"=w190, "time"=w191) -> (w189:cluster{"date":string, "time":string})
      n69 = Bundle By Name(cluster="Scan Info", "delay"=w185, "operator"=w179, "Scan Mode"=w183, "location"=w188) -> (w182:T5)
    }
    frame #3 {
      w218 = 10
      n70 = Unbundle By Name(w204) -> ("RF Info"=w203:T25, "Patient Info"=w202:T26)
      n71 = Unbundle(w207) -> ("Digitizer (dB)"=w214:sgl, "Gain (dB)"=w213:sgl, "Atten (dB)"=w212:sgl)
      n72 = Negate(x=w213) -> (-x=w208:sgl)
      n73 = Compound Arithmetic op=ADD(w214, w208, w212) -> (w211:sgl)
      n74 = Multiply(x=w211, y=w218) -> (x*y=w216:sgl)
      n75 = Concatenate Strings("File Name In", ".eye") -> ()  [unwired: 1 out]
      n76 = Round To Nearest(number=w216) -> (nearest integer value=w215:sgl)
      n77 = global read "PatientGlobals.vi" "Patient ID"() -> (w205:string)
      n78 = Divide(x=w215, y=w218) -> (x/y=w217:sgl)
      n79 = Number To Fractional String(number=w217, precision (6)=i16 1) -> ()  [unwired: 3 out]
      n80 = Bundle By Name(cluster=w203, "RF file name"="File Name In") -> (w209:T25)
      n81 = Bundle By Name(cluster=w202, "ID"=w205) -> (w201:T26)
    }
    frame #4 {
      # "Special case for VisSonics Acquisition\nand array scans of human eye"
      n82 = Unbundle By Name(w231) -> ("Avg Num"=w230:i32, "Total Dig CH"=w221:i32)
      n83 = Unbundle By Name(w232) -> ("Patient ID"=w235:string)
      n84 = Unbundle By Name(w220) -> ("Focal Zones"=w224:i16)
      n85 = Unbundle By Name(w229) -> ("Tissue Type"=w228:T27, "Misc Info"=w227:T28)
      n86 = Equal?(x=w235, y="") -> (x = y?=w234:bool)
      n87 = case shown="True" w234 {
        tunnel: [w245 _] -> w238
        tunnel: [w248 _] -> w237
        tunnel: [w243 w250] -> w236
        tunnel: w232 -> [w249 _]
        frame False {
          n88 = Unbundle By Name(w249) -> ("Eye Selector"=w247:enum32{"Left", "Right"}, "Plane"=w248:i8, "Scan Location"=w244:enum32{"Radio Selection 1", "Radio Selection 2"})
          n89 = To Unsigned Byte Integer(number=w247) -> (unsigned 8bit integer=w246:u8)
          n90 = To Unsigned Byte Integer(number=w244) -> (unsigned 8bit integer=w243:u8)
          n91 = Increment(x=w246) -> (x+1=w245:u8)
        }
        frame True {
          n92 = global read "SwitchGlobals.vi" "PulseSpacing (us)"() -> (w250:sgl)
        }
      }
      n93 = call "XMT-RCV Params.vi"("Dig Channels"=w221, "Ann Array Params"=w220) -> ("# RCV"=w222:i16, "# XMIT"=w223:i16)  [unwired: 4 in, 4 out]
      n94 = Multiply(x=w240, y=1000) -> (x*y=w239:sgl)
      n95 = Bundle By Name(cluster=w228, "organ"=w238, "disease type"=w237, "disease location"=w236) -> (w225:T27)
      n96 = Bundle By Name(cluster=w227, "avg num"=w230, "c speed"=w239, "Div By or SF zones"=w224, "XMIT CHS"=w223, "RCV CHS"=w222) -> (w226:T28)
    }
    frame #5 {
      # "Cross Axis Location"
      # "Main Axis Location"
      n97 = Unbundle By Name(w267) -> ("Add Axis"=w252:bool, "Global Position (mm)"=w264:dbl[], "scan pair"=w263:T8)
      n98 = case shown="\"Therapy With Scan\"..\"M Scan With Therapy Burst\"" w254 {
        tunnel: [TRUE FALSE] -> w251
        frame "Therapy With Scan".."M Scan With Therapy Burst" {
        }
        frame "1-D B Scan", Default {
        }
      }
      n99 = case shown="\"w-(x) scan\"..\"w-(z) scan\"" w263 {
        tunnel: w264 -> [w272 w275 w278 w281]
        tunnel: [w270 w273 w276 w279] -> w265
        frame "x-(y) scan", "x-(z) scan", "x-(w) scan", Default {
          n100 = Index Array(array=w272, index=0) -> (element=w270:dbl)
        }
        frame "y-(x) scan", "y-(z) scan", "y-(w) scan" {
          n101 = Index Array(array=w275, index=1) -> (element=w273:dbl)
        }
        frame "z-(x) scan", "z-(y) scan", "z-(w) scan" {
          n102 = Index Array(array=w278, index=2) -> (element=w276:dbl)
        }
        frame "w-(x) scan".."w-(z) scan" {
          n103 = Index Array(array=w281, index=3) -> (element=w279:dbl)
        }
      }
      n104 = case shown="\"y-(x) scan\", \"z-(x) scan\", \"w-(x) scan\", Default" w263 {
        tunnel: w264 -> [w284 w287 w290 w293]
        tunnel: [w282 w285 w288 w291] -> w266
        frame "y-(x) scan", "z-(x) scan", "w-(x) scan", Default {
          n105 = Index Array(array=w284, index=0) -> (element=w282:dbl)
        }
        frame "x-(y) scan", "z-(y) scan", "w-(y) scan" {
          n106 = Index Array(array=w287, index=1) -> (element=w285:dbl)
        }
        frame "y-(z) scan", "x-(z) scan", "w-(z) scan" {
          n107 = Index Array(array=w290, index=2) -> (element=w288:dbl)
        }
        frame "x-(w) scan".."z-(w) scan" {
          n108 = Index Array(array=w293, index=3) -> (element=w291:dbl)
        }
      }
      n109 = expression code="x*1e3"(w265) -> (w257:dbl)
      n110 = expression code="x*1e3"(w266) -> (w262:dbl)
      n111 = Or(x=w251, y=w252) -> (x .or. y?=w253:bool)
      n112 = Select(t=w257, s=w253, f=0.0) -> (s? t:f=w256:dbl)
      n113 = Bundle By Name(cluster=w261, "Xmit angle"=w262) -> (w260:T28)
      n114 = Bundle By Name(cluster=w259, "PSA"=w256) -> (w258:T26)
    }
    frame #6 {
      n115 = global read "PulserGlobals.vi" "Therapy Settings"() -> (w299:T29)
      n116 = Unbundle By Name(w295) -> ("Therapy Parameters"=w294:T30)
      n117 = Unbundle By Name(w301) -> ("Pre-Looks"=w300:i32)
      n118 = Unbundle By Name(w299) -> ("Therapy frequency (MHz)"=w298:dbl, "time therapy on (s)"=w297:dbl, "Therapy amplitude (mV)"=w296:dbl)
      n119 = Bundle By Name(cluster=w294, "Theraputic Freq (MHz)"=w298, "Time on (s)"=w297, "Therapy amplitude (mV)"=w296, "Lines Before"=w300) -> (w302:T30)
    }
    frame #7 {
      (unwired) TRUE
      n120 = global read "PatientGlobals.vi" "Node Info"() -> (w306:T31)
      n121 = Unbundle By Name(w306) -> ("Patient Number"=w305:u32)
      n122 = Unbundle By Name(w309) -> ("First Name"=w312:string, "Last Name"=w311:string, "Notes"=w307:string)
      n123 = Number To Decimal String(number=w305) -> (decimal integer string=w303:string)  [unwired: 1 in]
      n124 = Select(t=w303, s=w304, f=w307) -> (s? t:f=w308:string)
      n125 = Bundle("First Name"=w312, "Last Name"=w311, "Notes"=w308) -> (w310:T33)  [unwired: 1 in]
    }
  }
  n126 = Bundle By Name(cluster=w12, "header info"=w34, "A/D info"=w33, "Tranducer Info"=w30, "Scan Info"=w28, "Time/Date Info"=w31, "RF Info"=w25, "Patient Info"=w23, "Tissue Type"=w22, "Votage scaling"=w7, "Comment"=w8, "Misc Info"=w9, "Therapy Parameters"=w10, "Scan Settings"=w11, "Compression Parameters"=w20, "Patient Info Xtra"=w18) -> (w27:T14)
  "Header Out" <- w27
  n127 = call "MakeHeader.vi"("Header In"=w27) -> ("Header String"=→"Header String Out":string)  [unwired: 6 out]
